vi "InputUniv-Entry.vi"() -> (0 "정지 버튼 2":bool, 1 "확인 버튼 2":bool, 2 "엔트리번호출력":string, 3 "대학명출력":string)   [LabVIEW 2015]
panel:
  in  "정지 버튼":bool
  in  "엔트리번호":u8
  in  "확인 버튼":bool
  in  "대학명":string
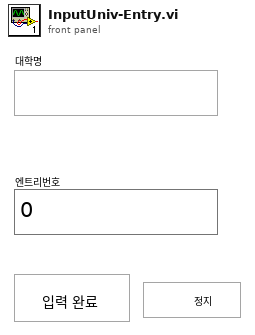
[diagram p1: front panel]
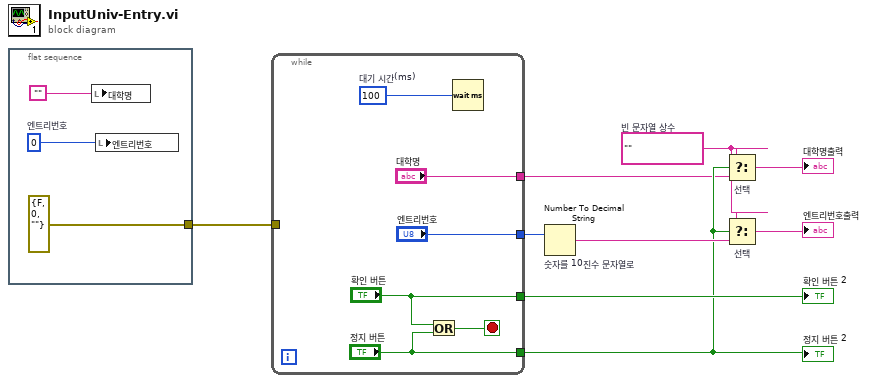
[diagram p0: block diagram]
diagram:
  w1 = ""  # 빈 문자열 상수
  n1 = flat-sequence {
    tunnel: [errorcluster {"status"=FALSE, "code"=0, "source"=""} ("에러 상수")] -> w9
    frame #0 {
      w10 = u8 0  # 엔트리번호
      n2 = local write "대학명"("") -> ()
      n3 = local write "엔트리번호"(w10) -> ()
    }
  }
  n4 = while {
    tunnel: ["대학명"] -> w3
    tunnel: ["엔트리번호"] -> w8
    tunnel: w9 -> [_]
    tunnel: ["확인 버튼"] -> w7
    tunnel: ["정지 버튼"] -> w4
    stop <- w14 stop-if-true
    w18 = u32 100  # 대기 시간(ms)
    n5 = Or(x="확인 버튼", y="정지 버튼") -> (x .or. y?=w14:bool)
    n6 = Wait (ms)(milliseconds to wait=w18) -> ()  [unwired: 1 out]
  }
  "확인 버튼 2" <- w7
  "정지 버튼 2" <- w4
  n7 = Number To Decimal String "숫자를 10진수 문자열로"(number=w8) -> (decimal integer string=w6:string)  [unwired: 1 in]
  n8 = Select "선택"(t=w1, s=w4, f=w3) -> (s? t:f=→"대학명출력":string)
  n9 = Select "선택"(t=w1, s=w4, f=w6) -> (s? t:f=→"엔트리번호출력":string)
